vi "PV ActiveLine - Error.vi"(7 "String IN":string) -> (0 "Errortext":string, 1 "Errornumber":i32)   [LabVIEW 2013, in "PV ActiveLine.lvlib"]
doc: "The ERROR word is cancelled when read out. If the error persists, it is immediately set again."
uses:
  <instrlib>/PV ActiveLine/PV ActiveLine.lvlib
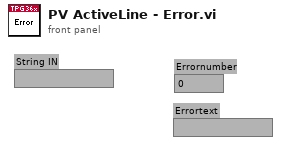
[diagram p1: front panel]
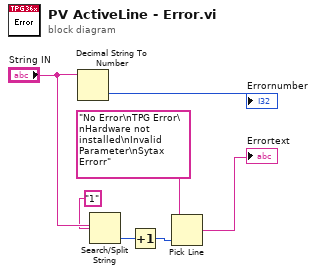
[diagram p0: block diagram]
diagram:
  n1 = Decimal String To Number(string="String IN") -> (number=→"Errornumber":i32)  [unwired: 2 in, 1 out]
  n2 = Search/Split String(string="String IN", search string/char (-)="1") -> (offset of match=w3:i32)  [unwired: 1 in, 2 out]
  n3 = Increment(x=w3) -> (x+1=w4:i32)
  n4 = Pick Line(multi-line string="No Error\nTPG Error\nHardware not installed\nInvalid Parameter\nSytax Errorr", line index=w4) -> (output string=→"Errortext":string)  [unwired: 1 in]
